vi "Layer Scan V3.vi"() -> ()   [LabVIEW 2024]
uses:
  <vilib>/DAQmx/write.llb/DAQmx Write (Analog 1D DBL NChan 1Samp).vi
  <vilib>/DAQmx/read.llb/DAQmx Read (Analog Wfm 1Chan NSamp).vi
  <vilib>/DAQmx/create/channels.llb/DAQmx Create Channel (AO-Voltage-Basic).vi
  <vilib>/DAQmx/create/channels.llb/DAQmx Create Channel (AI-Voltage-Basic).vi
  <vilib>/DAQmx/configure/timing.llb/DAQmx Timing (Sample Clock).vi
  <vilib>/DAQmx/miscellaneous.llb/DAQmx Fill In Error Info.vi
  <vilib>/express/express analysis/Spectral/Block/exnSpectralBlock spectral measurements RMS poly.vi
  <vilib>/express/express analysis/Spectral/Block/exnSpectralBlock spectral measurements RMS WFM.vi
  <vilib>/express/express analysis/Spectral/XNode/ExpressSpectralMeasurementsBlockNode.xnode
panel:
  out "FFT - (RMS)":cluster{"f0":dbl, "df":dbl, "magnitude":dbl[]}
  out "decimated array 2":dbl[](array[numeric])
  out "decimated array":dbl[](array[numeric])
  out "Y coord filename":i32
  out "x coord file name":i32
  out "Filename Out":path
  out "data AQ":waveform(dbl)(graph)
  in  "rate":dbl=1000.0 format="%0.2f"
  in  "samples per channel":i32=1000
  in  "Data File Name":path
  in  "Data folder Path":path
  in  "X offset":dbl
  in  "Y offset":dbl
  in  "distance":dbl
  in  "Y Count":dbl
  in  "X Count":dbl
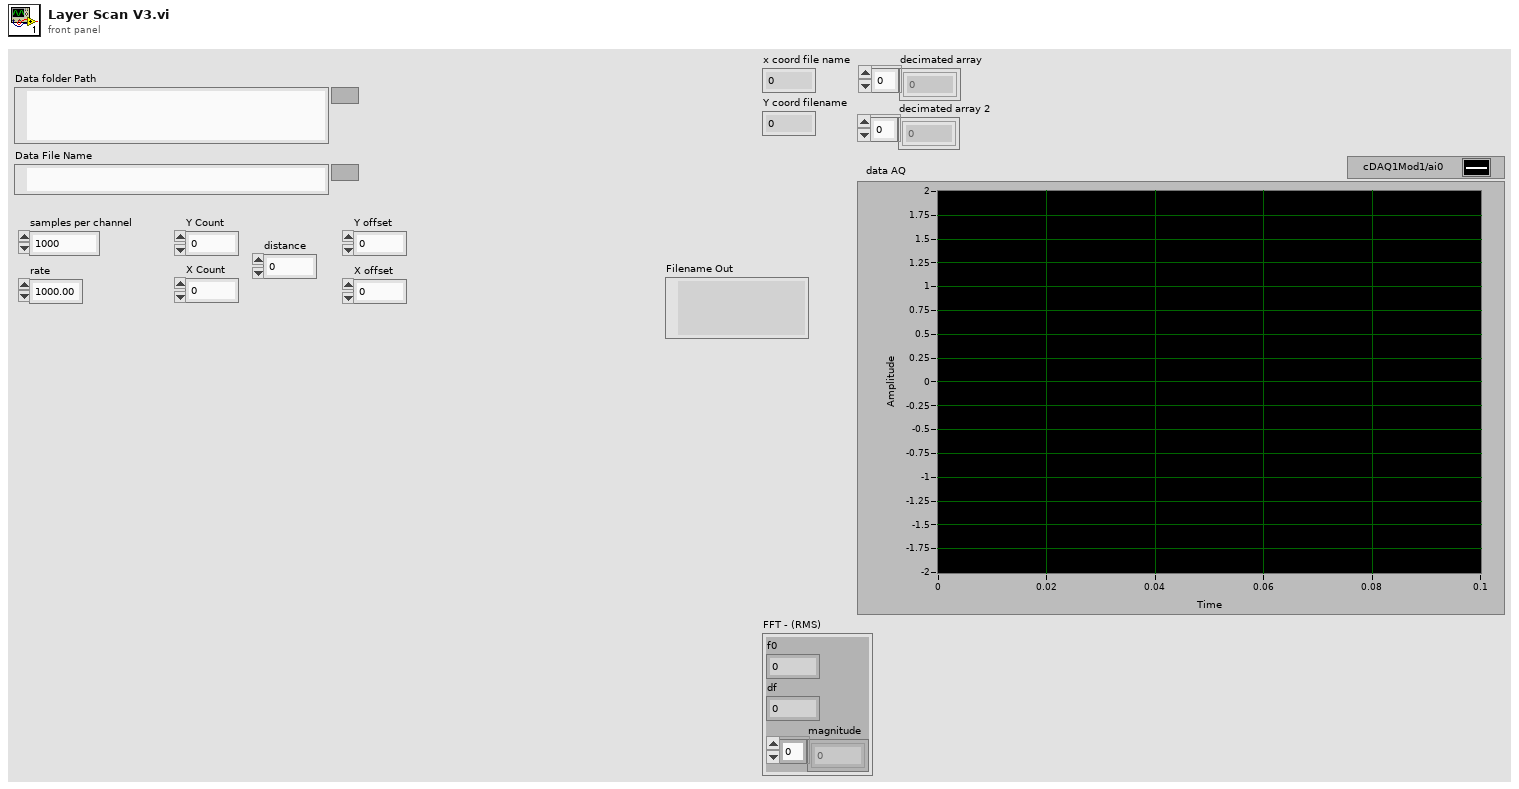
[diagram p1: front panel]
types:
  T1 = cluster{"averaging mode":u16, "weighting mode":u16, "number of averages":u32}
  T2 = cluster{"dB On (F)":bool, "unwrap phase (F)":bool, "convert to degree (F)":bool}
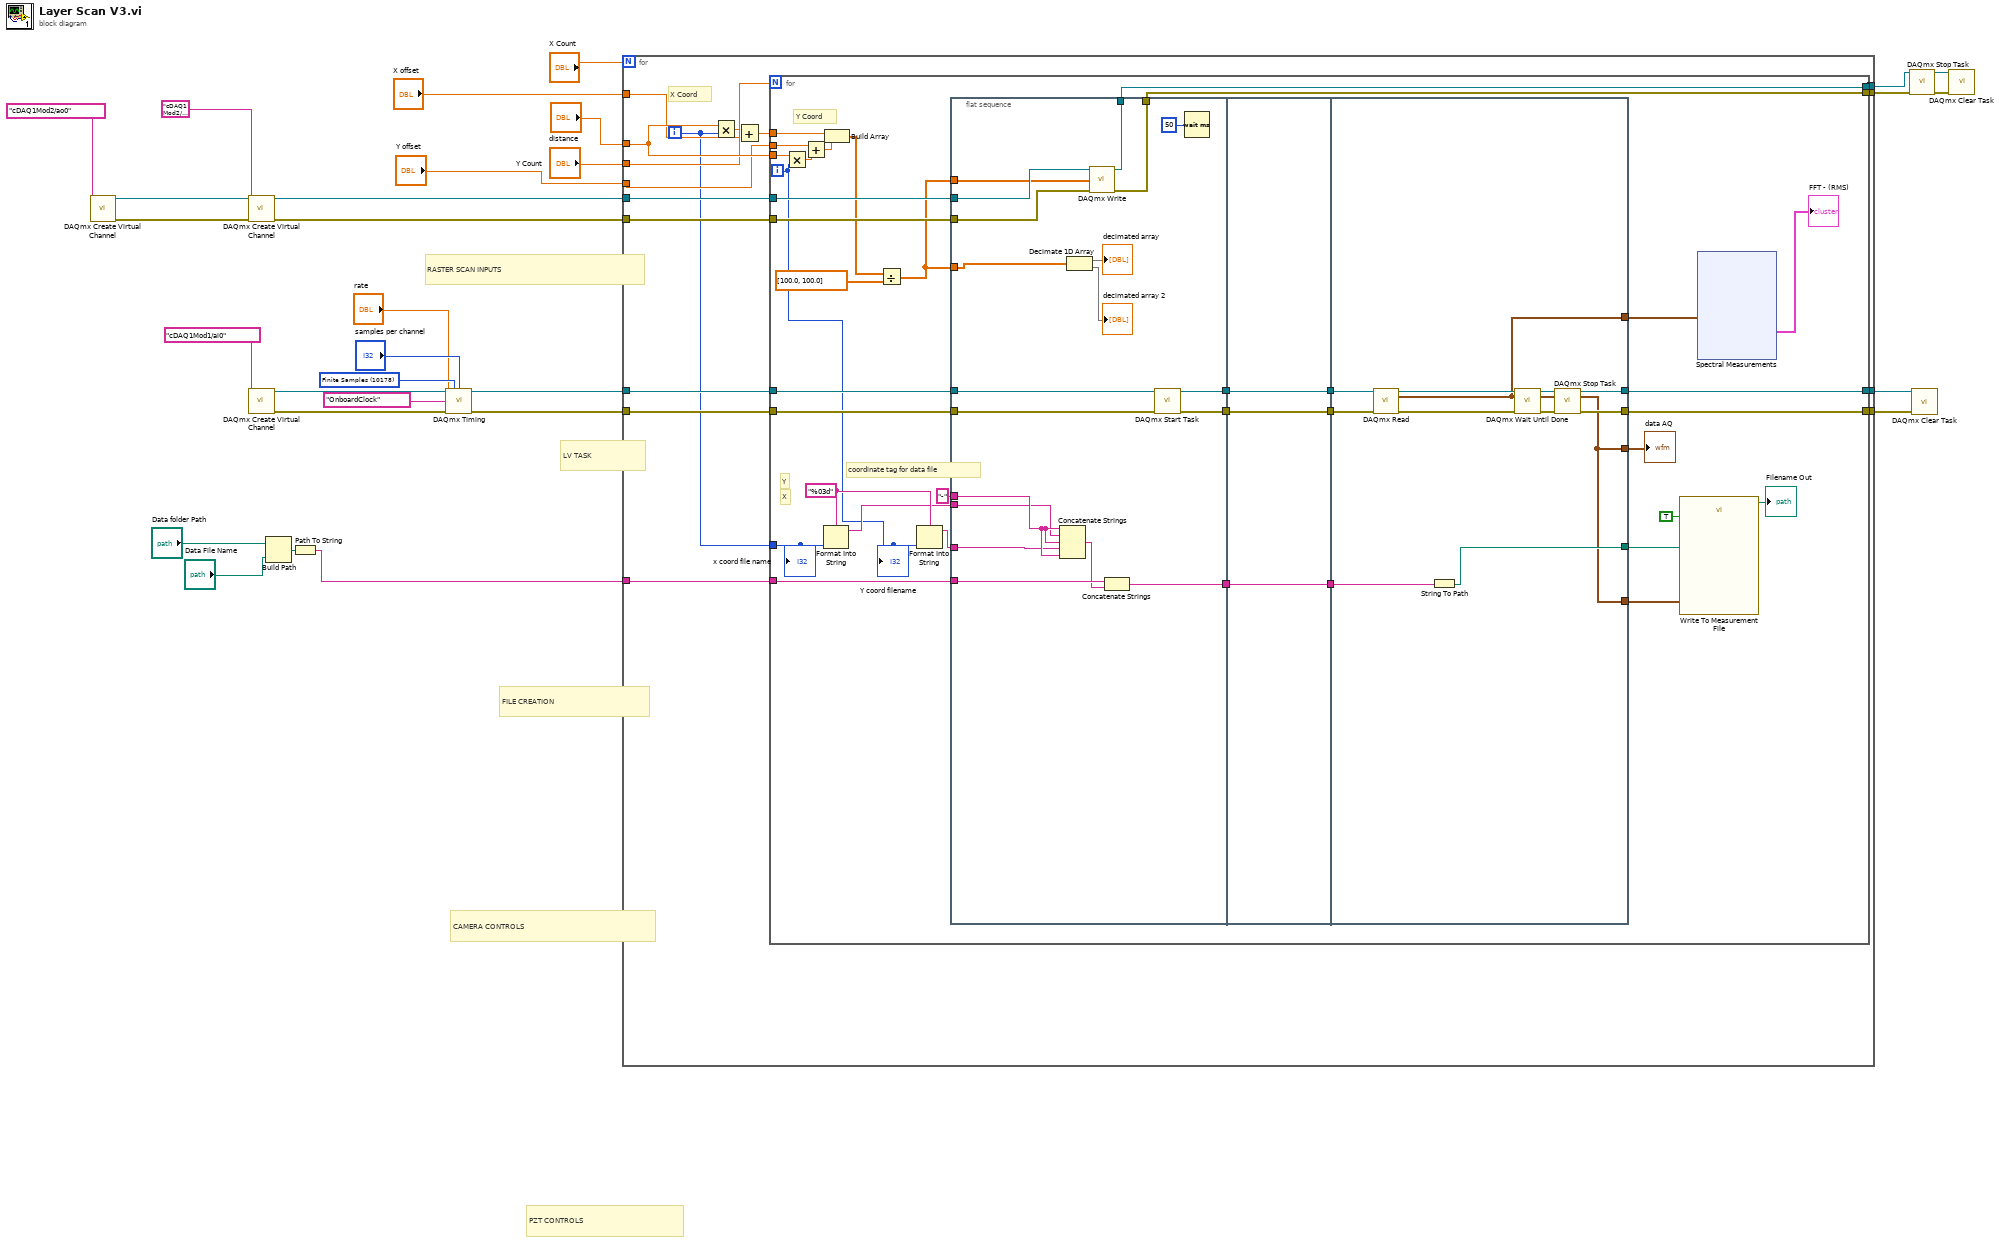
[diagram p0: block diagram]
diagram:
  w5 = 10178 items=["Finite Samples"=10178, "Continuous Samples"=10123, "Hardware Timed Single Point"=12522] ("sample mode")
  # "FILE CREATION"
  # "PZT CONTROLS"
  # "CAMERA CONTROLS"
  # "LV TASK"
  # "RASTER SCAN INPUTS"
  n1 = call-poly <vilib>:"DAQmx Create Virtual Channel.vi"("physical channels"=tag "cDAQ1Mod2/ao0") -> ("task out"=w23:refnum<k21>, "error out"=w22:errorcluster)  [unwired: 13 in]
  n2 = call-poly <vilib>:"DAQmx Create Virtual Channel.vi"("task in"=w23, "physical channels"=tag "cDAQ1Mod2/ao1", "error in"=w22) -> ("task out"=w21:refnum<k21>, "error out"=w20:errorcluster)  [unwired: 11 in]
  n3 = call-poly <vilib>:"DAQmx Create Virtual Channel.vi"("physical channels"=tag "cDAQ1Mod1/ai0") -> ("task out"=w15:refnum<k21>, "error out"=w14:errorcluster)  [unwired: 13 in]
  n4 = Build Path(base path="Data folder Path", name or relative path="Data File Name") -> (appended path=w7:path)
  n5 = Path To String(path=w7) -> (string=w6:string)
  n6 = call-poly <vilib>:"DAQmx Timing.vi"("task/channels in"=w15, "sample mode"=w5, "samples per channel"="samples per channel", "rate"="rate", "source"=tag "OnboardClock", "error in"=w14) -> ("task out"=w13:refnum<k21>, "error out"=w12:errorcluster)  [unwired: 8 in]
  n7 = for {
    N: "X Count" -> [_]
    tunnel: "distance" -> [w46]
    tunnel: "Y Count" -> [w45]
    tunnel: "Y offset" -> [w44]
    tunnel: "X offset" -> [w42]
    tunnel: w21 -> [w40]
    tunnel: w20 -> [w39]
    tunnel: [w38] -> w19
    tunnel: [w37] -> w18
    tunnel: w13 -> [w36]
    tunnel: w12 -> [w35]
    tunnel: [w34] -> w11
    tunnel: [w33] -> w10
    tunnel: w6 -> [w32]
    i -> [w31]
    # "X Coord"
    n8 = Multiply(x=w46, y=w31) -> (x*y=w43:dbl)
    n9 = Add(x=w43, y=w42) -> (x+y=w41:dbl)
    n10 = for {
      N: w45 -> [_]
      tunnel: w46 -> [w82]
      tunnel: w44 -> [w80]
      tunnel: w41 -> [w79]
      tunnel: w40 -> [w77]
      tunnel: w39 -> [w76]
      tunnel: [w74] -> w38
      tunnel: [w73] -> w37
      tunnel: w36 -> [w72]
      tunnel: w35 -> [w71]
      tunnel: [w70] -> w34
      tunnel: [w69] -> w33
      tunnel: w32 -> [w64]
      tunnel: w31 -> [w51]
      i -> [w50]
      w68 = "%03d" ("format string")
      # "coordinate tag for data file"
      # "X"
      # "Y"
      # "Y Coord"
      n11 = Multiply(x=w82, y=w50) -> (x*y=w81:dbl)
      n12 = Add(x=w80, y=w81) -> (x+y=w78:dbl)
      n13 = Format Into String(format string=w68, w51) -> (resulting string=w66:string)  [unwired: 2 in, 1 out]
      n14 = Build Array(w79, w78) -> (w75:dbl[])
      n15 = Divide(x=w75, y=dbl[] [100.0, 100.0]) -> (x/y=w49:dbl[])
      n16 = Format Into String(format string=w68, w50) -> (resulting string=w65:string)  [unwired: 2 in, 1 out]
      n17 = flat-sequence {
        tunnel: w77 -> [w110]
        tunnel: w76 -> [w109]
        tunnel: [w108] -> w74
        tunnel: [w107] -> w73
        tunnel: w72 -> [w106]
        tunnel: w71 -> [w105]
        tunnel: [w104] -> w63
        tunnel: [w103] -> w61
        tunnel: "-" ("string") -> [w102]
        tunnel: w66 -> [w101]
        tunnel: w65 -> [w100]
        tunnel: w64 -> [w99]
        tunnel: [w97] -> w59
        tunnel: w49 -> [w96]
        tunnel: w49 -> [w95]
        tunnel: w63 -> [w114]
        tunnel: [w114] -> w62
        tunnel: w61 -> [w113]
        tunnel: [w113] -> w60
        tunnel: w59 -> [w112]
        tunnel: [w112] -> w58
        tunnel: w62 -> [w125]
        tunnel: w60 -> [w124]
        tunnel: [w119] -> w70
        tunnel: [w118] -> w69
        tunnel: w58 -> [w117]
        tunnel: [w115] -> w57
        tunnel: [w115] -> w56
        tunnel: [w116] -> w55
        tunnel: [w115] -> w48
        frame #0 {
          n18 = Concatenate Strings(w102, w101, w102, w100, w102) -> (w98:string)
          n19 = Decimate 1D Array(w95) -> (→"decimated array":dbl[], →"decimated array 2":dbl[])
          n20 = call-poly <vilib>:"DAQmx Write.vi"("task/channels in"=w110, "data"=w96, "error in"=w109) -> ("task out"=w108:refnum<k21>, "error out"=w107:errorcluster)  [unwired: 10 in, 1 out]
          n21 = Concatenate Strings(w99, w98) -> (w97:string)
          n22 = call <vilib>:"DAQmx Start Task.vi"("task/channels in"=w106, "error in"=w105) -> ("task out"=w104:refnum<k21>, "error out"=w103:errorcluster)  [unwired: 12 in]
          n23 = Wait (ms)(milliseconds to wait=u32 50) -> ()  [unwired: 1 out]
        }
        frame #1 {
        }
        frame #2 {
          n24 = call-poly <vilib>:"DAQmx Read.vi"("task/channels in"=w125, "error in"=w124) -> ("task out"=w123:refnum<k21>, "data"=w115:waveform(dbl), "error out"=w122:errorcluster)  [unwired: 11 in]
          n25 = String To Path(string=w117) -> (path=w116:path)
          n26 = call <vilib>:"DAQmx Wait Until Done.vi"("task/channels in"=w123, "error in"=w122) -> ("task out"=w121:refnum<k21>, "error out"=w120:errorcluster)  [unwired: 12 in]
          n27 = call <vilib>:"DAQmx Stop Task.vi"("task/channels in"=w121, "error in"=w120) -> ("task out"=w119:refnum<k21>, "error out"=w118:errorcluster)  [unwired: 12 in]
        }
      }
      n28 = call "Write To Measurement File"("Signals"=w56, "Enable"=TRUE, "Filename"=w55) -> ("Filename Out"=→"Filename Out":path)  [unwired: 14 in, 2 out]
      n29 = xnode "Spectral Measurements"("Signals"=w48) -> ("FFT - (RMS)"=→"FFT - (RMS)":cluster{"f0":dbl, "df":dbl, "magnitude":dbl[]})  [unwired: 1 in, 2 out]
      "data AQ" <- w57
      "x coord file name" <- w51
      "Y coord filename" <- w50
    }
  }
  n30 = call <vilib>:"DAQmx Stop Task.vi"("task/channels in"=w19, "error in"=w18) -> ("task out"=w17:refnum<k21>, "error out"=w16:errorcluster)  [unwired: 12 in]
  n31 = call <vilib>:"DAQmx Clear Task.vi"("task in"=w11, "error in"=w10) -> ()  [unwired: 13 in, 1 out]
  n32 = call <vilib>:"DAQmx Clear Task.vi"("task in"=w17, "error in"=w16) -> ()  [unwired: 13 in, 1 out]
